vi "Command Type.vi"(11 "Transition Command Config in":refnum<class "Transition Command Config.lvclass">) -> (2 "Command Type":string)   [LabVIEW 2020, in "VolatusSeqConfig.lvlib" / "Transition Command Config.lvclass"]
uses:
  Transition Command Config.lvclass
  Transition Command Config.lvclass/Transition Command Config.ctl
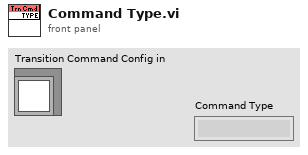
[diagram p1: front panel]
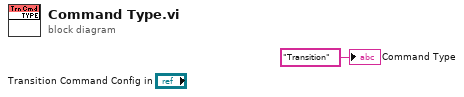
[diagram p0: block diagram]
diagram:
  "Command Type" <- "Transition" ("Command Type")
